vi "Continuous GPS WP List Record+.vi"(10 "Read Point?":bool) -> (3 "Saved?":bool)   [LabVIEW 2009]
uses:
  Functional Global Variables/Actions for FG's.ctl
  Remote Control/Motor Command.ctl
  <vilib>/Platform/TimedLoop/XDataNode/wakeup.ctl
  <vilib>/Platform/TimedLoop/XDataNode/XDNodeRunTimeDep.lvlib
  <vilib>/Platform/TimedLoop/XDataNode/nitl_modes.ctl
  <vilib>/Platform/TimedLoop/XDataNode/timing_clust.ctl
  <vilib>/Platform/TimedLoop/XDataNode/XDataNode.xnode
  TypeDefs/Queue TypeDefs/Motor State.ctl
  TypeDefs/Queue TypeDefs/Motor Instruction.ctl
  <vilib>/Platform/TimedLoop/XDataNode/loadlvalarms.vi
panel:
  out "Array":cluster{"Longitude":dbl, "Latitude":dbl}[](array[cluster]) {"Longitude" format="%#_14g"; "Latitude" format="%#_14g"}
  in  "stop":bool
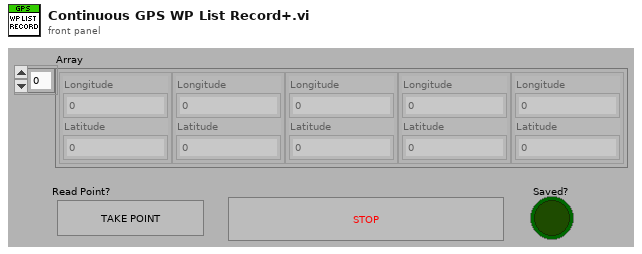
[diagram p1: front panel]
types:
  T1 = enum16{"open", "replace", "create", "open or create", "replace or create", "replace or create with confirmation"}
  T2 = typedef "Motor Instruction.ctl" = cluster{"Motor State":T3, "Motor Command":T4}
  T3 = typedef "Motor State.ctl" = enum16{"Wait", "Initialize", "Check FET", "Run", "Stop"}
  T4 = typedef "Motor Command.ctl" = cluster{"Speed":i16, "Turn":i16}
  T5 = typedef "Actions for FG's.ctl" = enum16{"Read", "Write"}
  T6 = typedef "XDNodeRunTimeDep.lvlib/timing_clust.ctl" = cluster{"Expected End [f-1]":u64, "Actual End [f-1]":u64, "Finished Late? [f-1]":bool, "Expected End [i-1]":u64, "Actual End [i-1]":u64, "Finished Late? [i-1]":bool, "Expected Start [i]":u64, "Actual Start [i]":u64, "Expected Start [f]":u64, "Actual Start [f]":u64, "Source Name":string, "Structure Name":string, "Period":i64, "Deadline":i64, "Offset":i64, "Start":i64, "Priority":i32, "Timeout":i32, "Mode":T7, "Wakeup Reason":T8, "Error":errorcluster, "Source Type":string, "Secondary Source Type":string, "Global End Time":u64, "Global Start Time":u64, "Frame Duration":u64, "Iteration Duration":u64, "Assigned CPU":i32, "I/O Scan Engine Mode":u32}
  T7 = typedef "XDNodeRunTimeDep.lvlib/nitl_modes.ctl" = enum32{"No Change", "Process missed periods, maintain original phase", "Discard missed periods, maintain original phase", "Process missed periods, ignore original phase", "Discard missed periods, ignore original phase"}
  T8 = typedef "XDNodeRunTimeDep.lvlib/wakeup.ctl" = enum32{"Normal", "Aborted", "Asynchronous wakeup", "Timing source error", "Timed loop error", "Timeout"}
  T9 = typedef "GPS Data.ctl" = cluster{"Latitude":dbl, "Longitude":dbl}
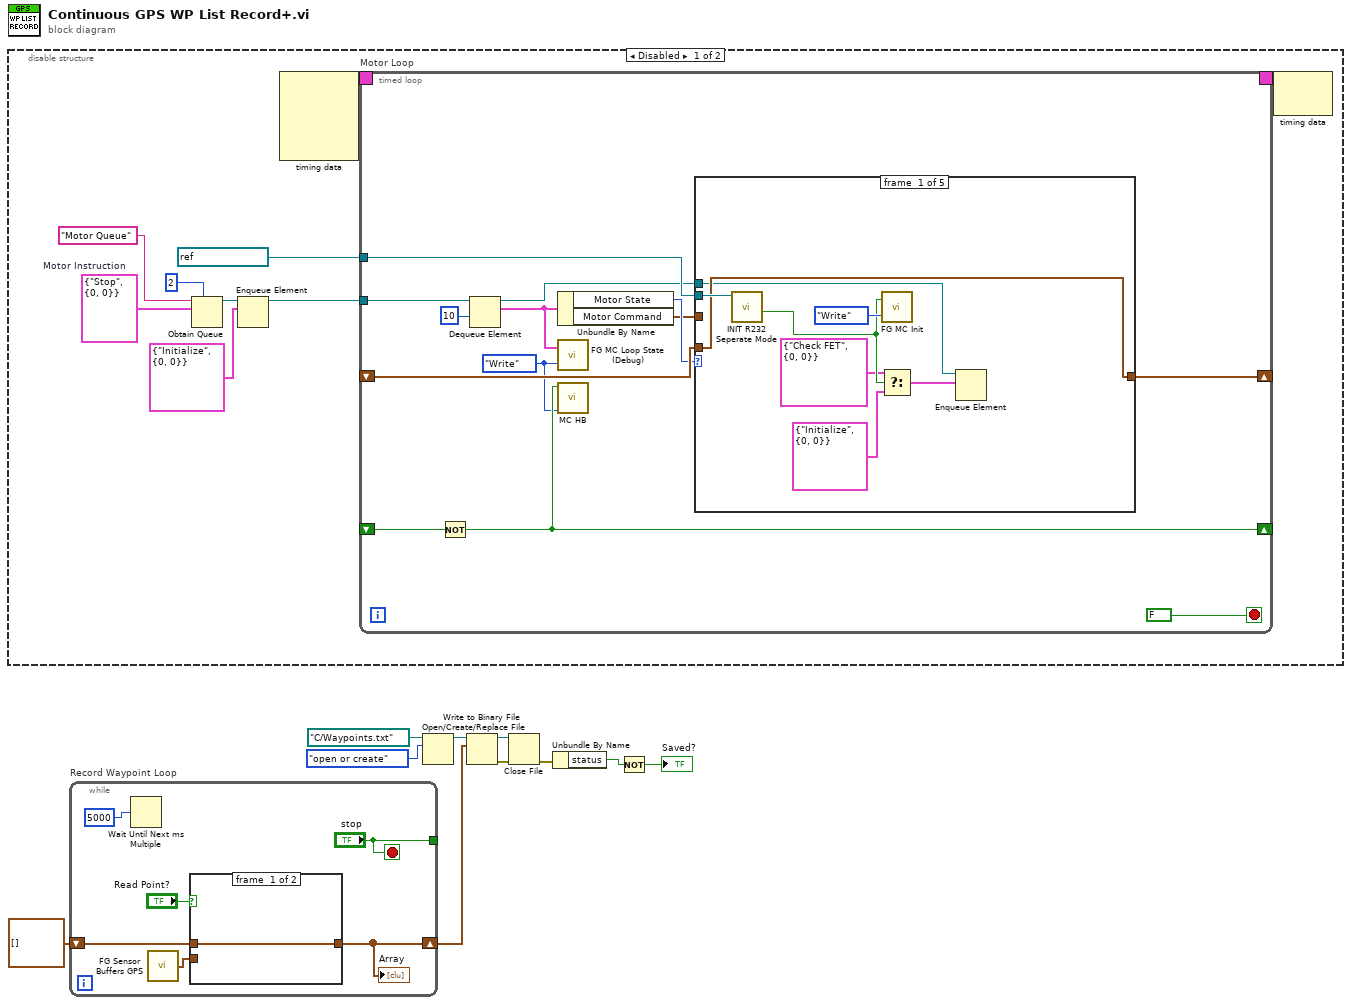
[diagram p0: block diagram]
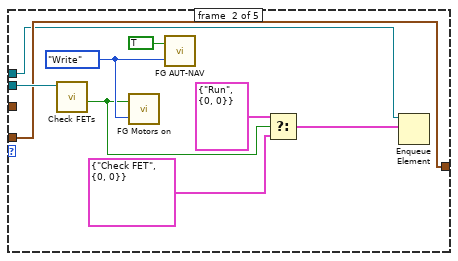
[diagram p2: hidden frame]
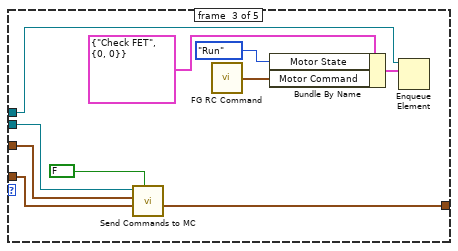
[diagram p3: hidden frame]
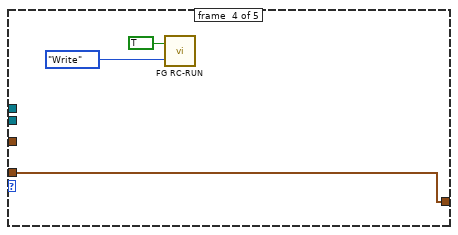
[diagram p4: hidden frame]
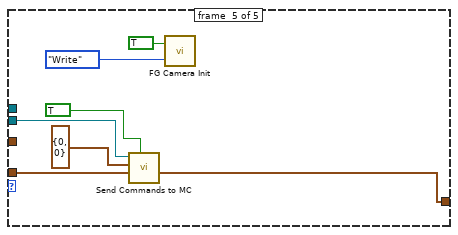
[diagram p5: hidden frame]
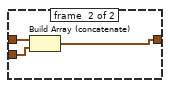
[diagram p7: hidden frame]
diagram:
  n1 = disable-structure shown="Disabled" {
    frame #0 {
      w16 = T2 {"Motor State"=enum."Stop", "Motor Command"={"Speed"=0, "Turn"=0}}  # Motor Instruction
      n2 = Obtain Queue(max queue size (-1, unlimited)=2, name (unnamed)="Motor Queue", element data type=w16) -> (queue out=w13:refnum<queue>)  [unwired: 2 in, 2 out]
      n3 = Enqueue Element(queue=w13, element=T2 {"Motor State"=enum."Initialize", "Motor Command"={"Speed"=0, "Turn"=0}}) -> (queue out=w12:refnum<queue>)  [unwired: 2 in, 2 out]
      n4 = node-c288() -> (w19:T6)  [unwired: 4 in]
      n5 = timed-loop "Motor Loop" {
        timing: w19 -> [_]
        timing-out: [_] -> w18
        shift-right: [w30] -> _
        shift-left: _ -> [w31]
        shift-right: [w27] -> _
        shift-left: _ -> [w29]
        tunnel: refnum<visa-resource-name> "RIO0::INSTR" ("MC VISA resource") -> [w28]
        tunnel: w12 -> [w22]
        stop <- FALSE stop-if-true
        w24 = Actions_for_FG's."Write" ("FG Action")
        n6 = Not(x=w29) -> (.not. x?=w27:bool)
        n7 = Dequeue Element(queue=w22, timeout in ms (-1)=10) -> (queue out=w20:refnum<queue>, element=w23:T2)  [unwired: 1 in, 2 out]
        n8 = Unbundle By Name(w23) -> ("Motor State"=w26:T3, "Motor Command"=w25:T4)
        n9 = call "FG MC Loop State (Debug).vi"("FG Action (Read)"=w24, "Motor Instruction in"=w23) -> ()  [unwired: 1 out]
        n10 = call "MC HB.vi"("FG Action"=w24, "MC HB in"=w27) -> ()  [unwired: 9 in, 1 out]
        n11 = case shown="\"Initialize\"" w26 {
          tunnel: w28 -> [w40 w49 w59 _ w69]
          tunnel: w25 -> [_ _ w57 _ _]
          tunnel: w31 -> [w39 w48 w56 w62 w65]
          tunnel: [w39 w48 w55 w62 w66] -> w30
          tunnel: w20 -> [w33 w44 w50 _ _]
          frame #0 {
            n12 = call "INIT R232 Seperate Mode.vi"("MC VISA resource in"=w40) -> ("MC Init Complete"=w37:bool)  [unwired: 8 in, 2 out]
            n13 = call "FG MC Init.vi"("FG Action"=Actions_for_FG's."Write", "MC Init in"=w37) -> ()  [unwired: 1 out]
            n14 = Select(t=T2 {"Motor State"=enum."Check FET", "Motor Command"={"Speed"=0, "Turn"=0}} ("element"), s=w37, f=T2 {"Motor State"=enum."Initialize", "Motor Command"={"Speed"=0, "Turn"=0}} ("element")) -> (s? t:f=w36:T2)
            n15 = Enqueue Element(queue=w33, element=w36) -> ()  [unwired: 2 in, 3 out]
          }
          frame #1 {
            w47 = Actions_for_FG's."Write" ("FG Action")
            n16 = call "Check FETs.vi"("MC VISA resource in"=w49) -> ("FETs on?"=w41:bool)  [unwired: 6 in, 4 out]
            n17 = call "FG Motors on.vi"("FG Action"=w47, "Motors on ? in"=w41) -> ()  [unwired: 1 out]
            n18 = call "FG AUT-NAV.vi"("FG Action (Read)"=w47, "Aut/!Nav in"=TRUE) -> ()  [unwired: 1 in, 1 out]
            n19 = Select(t=T2 {"Motor State"=enum."Run", "Motor Command"={"Speed"=0, "Turn"=0}} ("element"), s=w41, f=T2 {"Motor State"=enum."Check FET", "Motor Command"={"Speed"=0, "Turn"=0}} ("element")) -> (s? t:f=w45:T2)
            n20 = Enqueue Element(queue=w44, element=w45) -> ()  [unwired: 2 in, 3 out]
          }
          frame #2 {
            n21 = call "Send Commands to MC.vi"("Pause Motors"=FALSE, "Prev MC cmd"=w56, "Motor Command"=w57, "MC refrence in"=w59) -> ("New MC cmd"=w55:cluster{"cmd a":i16, "cmd b":i16})  [unwired: 4 in, 3 out]
            n22 = call "FG RC Command.vi"() -> ("Motor Command out"=w53:T4)  [unwired: 2 in]
            n23 = Bundle By Name(cluster=T2 {"Motor State"=enum."Check FET", "Motor Command"={"Speed"=0, "Turn"=0}} ("element"), "Motor State"=Motor_State."Run", "Motor Command"=w53) -> (w51:T2)
            n24 = Enqueue Element(queue=w50, element=w51) -> ()  [unwired: 2 in, 3 out]
          }
          frame #3 {
            n25 = call "FG RC-RUN.vi"("FG Action (Read)"=Actions_for_FG's."Write", "RC/!Run in"=TRUE) -> ()  [unwired: 1 in, 1 out]
          }
          frame #4 {
            n26 = call "Send Commands to MC.vi"("Pause Motors"=TRUE, "Prev MC cmd"=w65, "Motor Command"=T4 {"Speed"=0, "Turn"=0}, "MC refrence in"=w69) -> ("New MC cmd"=w66:cluster{"cmd a":i16, "cmd b":i16})  [unwired: 4 in, 3 out]
            n27 = call "FG Camera Init.vi"("FG Action"=Actions_for_FG's."Write", "Camera Init in"=TRUE) -> ()  [unwired: 1 out]
          }
        }
      }
      n28 = node-c288(w18) -> ()  [unwired: 1 out]
    }
    frame #1 {
    }
  }
  n29 = while "Record Waypoint Loop" {
    shift-right: [w79] -> w8
    shift-left: cluster{"Longitude":dbl, "Latitude":dbl}[] [] -> [w78]
    tunnel: ["stop"] -> _
    stop <- "stop" stop-if-true
    n30 = Wait Until Next ms Multiple(millisecond multiple=u32 5000 ("millisecond timer value")) -> ()  [unwired: 1 out]
    n31 = call "FG Sensor Buffers GPS.vi"() -> ("GPS Buffer out"=w77:T9)  [unwired: 2 in]
    n32 = case shown="True" "Read Point?" {
      tunnel: w78 -> [w80 w83]
      tunnel: [w80 w82] -> w79
      tunnel: w77 -> [_ w81]
      frame #0 {
      }
      frame #1 {
        n33 = Build Array (concatenate)(w83, w81) -> (w82:T9[])
      }
    }
    "Array" <- w79
  }
  n34 = Open/Create/Replace File(file path (use dialog)=path "C:/Waypoints.txt", operation (0:open)=T1."open or create") -> (refnum out=w7:refnum<file>)  [unwired: 4 in, 2 out]
  n35 = Write to Binary File(file (use dialog)=w7, data=w8) -> (refnum out=w6:refnum<file>, error out=w5:errorcluster)  [unwired: 4 in, 1 out]
  n36 = Close File(refnum=w6, error in=w5) -> (error out=w3:errorcluster)  [unwired: 1 out]
  n37 = Unbundle By Name(w3) -> ("status"=w2:bool)
  n38 = Not(x=w2) -> (.not. x?=→"Saved?":bool)
